vi "Initialise.vi"(8 "error in (no error)":errorcluster, 10 "Message in":refnum<class "InitialiseMessage.lvclass">, 11 "DAQMH121119OrcaFlash in":refnum<class "DAQOrcaFlash.lvclass">) -> (0 "error out":errorcluster, 3 "DAQMH121119OrcaFlash out":refnum<class "DAQOrcaFlash.lvclass">)   [LabVIEW 2012, in "DAQOrcaFlash.lvclass"]
doc: "This member function is called when the statemachine in the run.vi receives an 'initialise' message. It mainly initialises the RabbitMQ connectivity. \n\nOverride this member function in your derived class to initialise hardware or software resources (but don't forget to call the parent method). If your component owns subcomponents, they count as resources, so you have to initialise them by calling their own initialise functions."
uses:
  DAQOrcaFlash.lvclass
  <vilib>/Distrio/Murmex/InitialiseMessage/InitialiseMessage.lvclass
  <vilib>/Distrio/Murmex/Murmex/Murmex.lvclass
  <vilib>/Distrio/Murmex/TerminateMessage/TerminateMessage.lvclass
  <vilib>/Distrio/Murmex/UpdateMessage/UpdateMessage.lvclass
  imaging_mode.ctl
  DAQOrcaFlash.lvclass/DAQOrcaFlash.ctl
  <vilib>/Distrio/Murmex/GenericMessage/GenericMessage.lvclass
  <vilib>/Distrio/Murmex/Message/Add or replace parameter.vi
panel:
  # "This method is called when the INTIALISE\ntrigger is sent. \n\nOverride this method when your component needs to\nrespond to this trigger. \n\nCall parent for proper implementation"
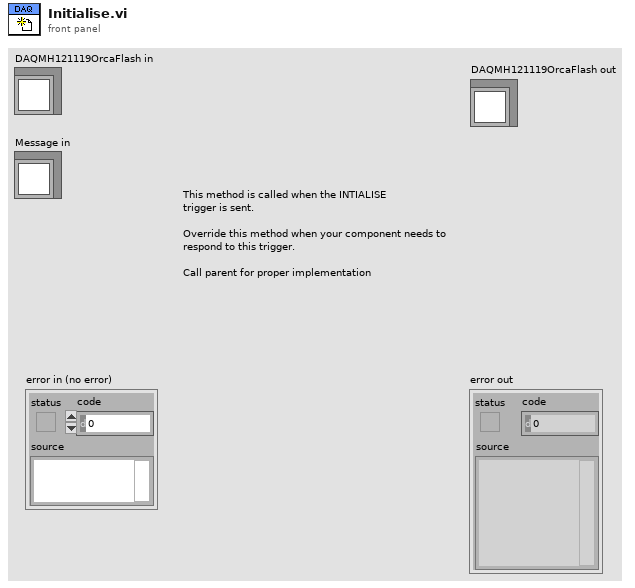
[diagram p1: front panel]
types:
  T1 = typedef "DAQOrcaFlash.lvclass/imaging_mode.ctl" = enum16{"focus mode", "single sweep"}
  T2 = cluster{"Mode":u32, "Polarity":u32, "Period":dbl, "Delay":dbl}
  T3 = typedef "Image Type" = u32
  T4 = typedef "IMAQ Image.ctl" = refnum<image>
  T5 = cluster{"height":u32, "width":u32, "datatype":u32}
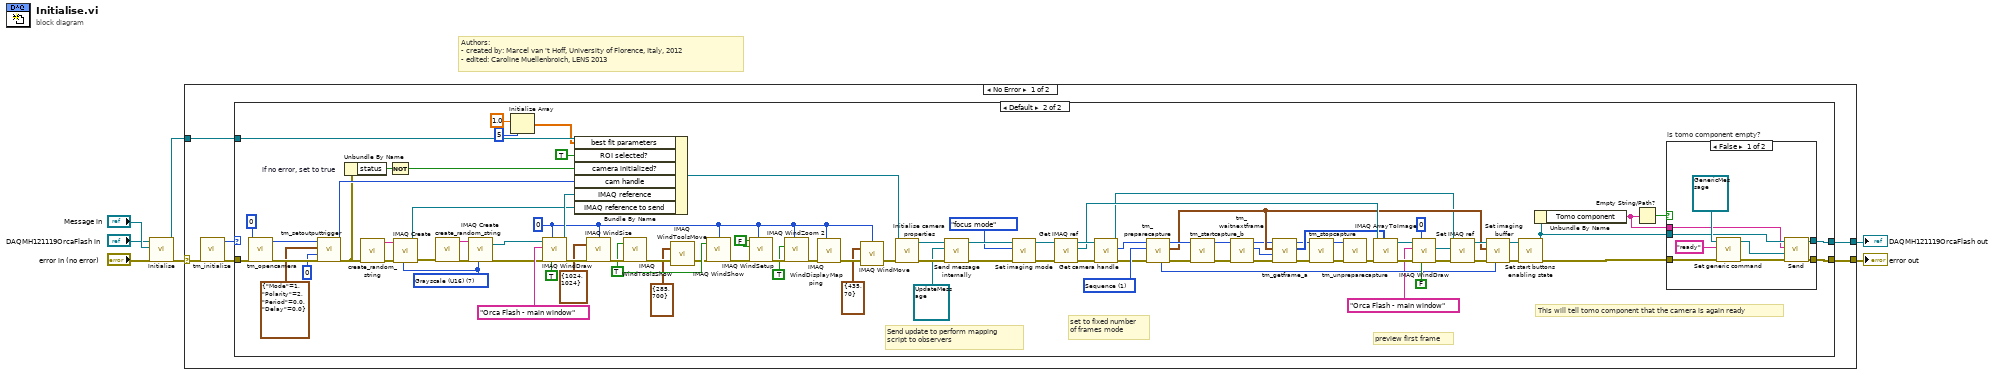
[diagram p0: block diagram]
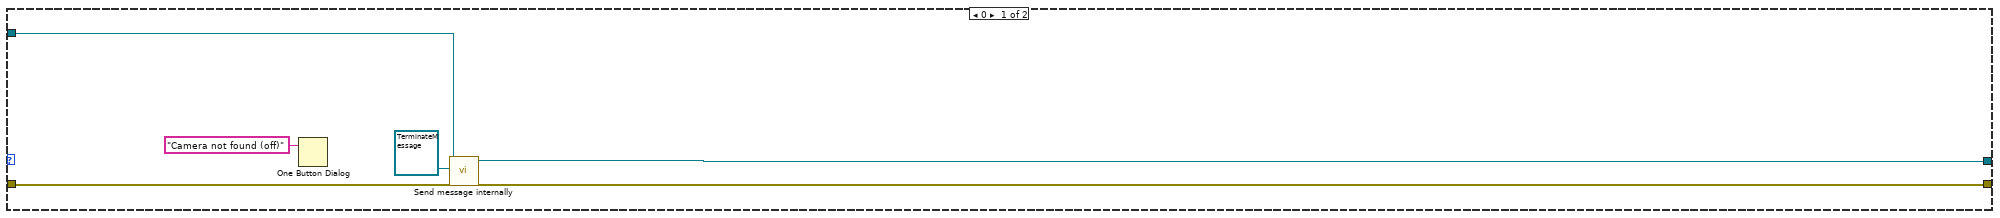
[diagram p2: hidden frame]
diagram:
  # "Authors: \n- created by: Marcel van 't Hoff, University of Florence, Italy, 2012\n- edited: Caroline Muellenbroich, LENS 2013"
  n1 = call-parent "Initialise.vi"("error in (no error)"="error in (no error)", "Message in"="Message in", "Murmex in"="DAQMH121119OrcaFlash in") -> ("error out"=w4:errorcluster, "Murmex out"=w3:refnum<class "DAQOrcaFlash.lvclass">)  [unwired: 7 in]
  n2 = case shown="No Error" w4 {
    selector: w4 -> [w12 w122]
    tunnel: w3 -> [w11 w123]
    tunnel: [w10 w123] -> w2
    tunnel: [w9 w122] -> w1
    frame No Error {
      n3 = call <userlib>:"tm_initialize.vi"("error in (no error)"=w12) -> ("error out"=w13:errorcluster, "Number Of Cameras"=w8:u32)  [unwired: 7 in, 2 out]
      n4 = case shown="Default" w8 {
        tunnel: w13 -> [w19 w110]
        tunnel: w11 -> [w17 w106]
        tunnel: [w16 w39] -> w10
        tunnel: [w18 w40] -> w9
        frame 0 {
          n5 = One Button Dialog(message="Camera not found (off)") -> ()  [unwired: 1 in, 1 out]
          n6 = call <vilib>:"Send message internally.vi"("error in (no error)"=w19, "Message"=refnum<class "TerminateMessage.lvclass"> refnum ("TerminateMessage"), "Murmex in"=w17) -> ("error out"=w18:errorcluster, "Murmex out"=w16:refnum<class "DAQOrcaFlash.lvclass">)  [unwired: 7 in]
        }
        frame Default {
          w68 = 1 items=["Snap", "Sequence"] ("Capture mode")
          w95 = FALSE ("Window can grow? (Yes)")
          w24 = 0 ("Window Number (0...15)")
          w97 = TRUE ("Hide/Show (Show)")
          w84 = T3 7 items=["Grayscale (U8)", "Grayscale (I16)", "Grayscale (SGL)", "Complex (CSG)", "RGB (U32)", "HSL (U32)", "RGB (U64)", "Grayscale (U16)"] ("Image Type")
          # "This will tell tomo component that the camera is again ready"
          # "preview first frame"
          # "set to fixed number\nof frames mode"
          # "Send update to perform mapping\nscript to observers"
          n7 = call <userlib>:"tm_opencamera.vi"("error in (no error)"=w110, "Camera Index"=u32 0) -> ("error out"=w91:errorcluster, "Handle out"=w92:u32)  [unwired: 7 in, 1 out]
          n8 = call <userlib>:"tm_setoutputtrigger.vi"("error in (no error)"=w91, "Index"=0, "Parameters"=T2 {"Mode"=1, "Polarity"=2, "Period"=0.0, "Delay"=0.0}, "Handle in"=w92) -> ("error out"=w78:errorcluster, "Handle out"=w88:u32)  [unwired: 6 in]
          n9 = Unbundle By Name "if no error, set to true"(w78) -> ("status"=w77:bool)
          n10 = call "create_random_string.vi"("error in (no error)"=w78) -> ("error out"=w85:errorcluster, "random string"=w83:string)  [unwired: 9 in]
          n11 = Not(x=w77) -> (.not. x?=w76:bool)
          n12 = call "IMAQ Create"("Image Name"=w83, "Image Type"=w84, "error in (no error)"=w85) -> ("New Image"=w82:T4, "error out"=w86:errorcluster)  [unwired: 2 in]
          n13 = call "create_random_string.vi"("error in (no error)"=w86) -> ("error out"=w108:errorcluster, "random string"=w107:string)  [unwired: 9 in]
          n14 = call "IMAQ Create"("Image Name"=w107, "Image Type"=w84, "error in (no error)"=w108) -> ("New Image"=w104:T4, "error out"=w101:errorcluster)  [unwired: 2 in]
          n15 = Initialize Array(1.0 ("element"), 5 ("dimension size")) -> (w33:dbl[])
          n16 = call "IMAQ WindDraw"("Resize to Image Size? (Y)"=TRUE, "Window Number (0...15)"=w24, "error in (no error)"=w101, "Title"="Orca Flash - main window", "Image"=w104) -> ("error out"=w100:errorcluster, "Image Out (duplicate)"=w105:T4)  [unwired: 5 in]
          n17 = Bundle By Name(cluster=w106, "best fit parameters"=w33, "ROI selected?"=TRUE ("Runtime cluster.ROI selected?"), "camera initialized?"=w76, "cam handle"=w88, "IMAQ reference"=w105, "IMAQ reference to send"=w82) -> (w87:refnum<class "DAQOrcaFlash.lvclass">)
          n18 = call "IMAQ WindSize"("error in (no error)"=w100, "Width & Height"=cluster{"Width":i32, "Height":i32} {"Width"=1024, "Height"=1024}, "Window Number"=w24) -> ("error out"=w99:errorcluster)  [unwired: 3 in, 2 out]
          n19 = call "IMAQ WindToolsShow"("Hide/Show (Show)"=w97, "error in (no error)"=w99) -> ("error out"=w22:errorcluster)  [unwired: 3 in, 1 out]
          n20 = call "IMAQ WindToolsMove"("Coordinates"=cluster{"X Position":i32, "Y Position":i32} {"X Position"=285, "Y Position"=700}, "error in (no error)"=w22) -> ("error out"=w21:errorcluster)  [unwired: 3 in, 1 out]
          n21 = call "IMAQ WindShow"("error in (no error)"=w21, "Hide/Show (Show)"=w97, "Window Number (0...15)"=w24) -> ("error out"=w96:errorcluster)  [unwired: 3 in, 2 out]
          n22 = call "IMAQ WindSetup"("Window Number (0...15)"=w24, "error in (no error)"=w96, "Window can close? (Yes)"=w95, "Window can grow? (Yes)"=w95) -> ("error out"=w94:errorcluster)  [unwired: 7 in]
          n23 = call "IMAQ WindZoom 2"("Window Number (0...15)"=w24, "error in (no error)"=w94, "Zoom to Fit? (False)"=TRUE) -> ("error out"=w75:errorcluster)  [unwired: 5 in, 3 out]
          n24 = call "IMAQ WindDisplayMapping"("Window Number (0...15)"=w24, "error in (no error)"=w75) -> ("error out"=w26:errorcluster)  [unwired: 8 in, 1 out]
          n25 = call "IMAQ WindMove"("Window Number (0...15)"=w24, "Coordinates (screen)"=cluster{"X Position":i32, "Y Position":i32} {"X Position"=435, "Y Position"=70}, "error in (no error)"=w26) -> ("error out"=w25:errorcluster)  [unwired: 2 in, 1 out]
          n26 = call-dynamic "Initialise camera properties.vi"("error in (no error)"=w25, "DAQOrcaFlash in"=w87) -> ("error out"=w81:errorcluster, "DAQOrcaFlash out"=w80:refnum<class "DAQOrcaFlash.lvclass">)  [unwired: 8 in]
          n27 = call <vilib>:"Send message internally.vi"("error in (no error)"=w81, "Message"=refnum<class "UpdateMessage.lvclass"> refnum ("Distrio Murmex 1.0:UpdateMessage"), "Murmex in"=w80) -> ("error out"=w44:errorcluster, "Murmex out"=w42:refnum<class "DAQOrcaFlash.lvclass">)  [unwired: 7 in]
          n28 = call "Set imaging mode.vi"("error in (no error)"=w44, "imaging mode"=imaging_mode."focus mode", "DAQMH121119OrcaFlash in"=w42) -> ("error out"=w45:errorcluster, "DAQMH121119OrcaFlash out"=w43:refnum<class "DAQOrcaFlash.lvclass">)  [unwired: 7 in]
          n29 = call "Get IMAQ ref.vi"("error in (no error)"=w45, "DAQMH121119OrcaFlash in"=w43) -> ("error out"=w73:errorcluster, "IMAQ reference"=w63:T4, "DAQMH121119OrcaFlash out"=w74:refnum<class "DAQOrcaFlash.lvclass">)  [unwired: 7 in]
          n30 = call "Get camera handle.vi"("error in (no error)"=w73, "DAQMH121119OrcaFlash in"=w74) -> ("error out"=w54:errorcluster, "cam handle"=w55:u32, "DAQMH121119OrcaFlash out"=w57:refnum<class "DAQOrcaFlash.lvclass">)  [unwired: 7 in]
          n31 = call <userlib>:"tm_preparecapture.vi"("error in (no error)"=w54, "Capture mode"=w68, "Handle in"=w55) -> ("error out"=w69:errorcluster, "Buffer Info"=w61:T5, "Handle out"=w67:u32, "Image type"=w60:u32)  [unwired: 5 in]
          n32 = call <userlib>:"tm_startcapture_b.vi"("error in (no error)"=w69, "Handle in"=w67) -> ("error out"=w66:errorcluster, "Handle out"=w46:u32)  [unwired: 8 in]
          n33 = call <userlib>:"tm_waitnextframe.vi"("error in (no error)"=w66, "Handle in"=w46) -> ("error out"=w53:errorcluster, "Frame Index"=w65:i32, "Handle out"=w52:u32)  [unwired: 6 in, 1 out]
          n34 = call <userlib>:"tm_getframe_a.vi"("error in (no error)"=w53, "Frame Index"=w65, "Buffer Info"=w61, "Handle in"=w52) -> ("error out"=w48:errorcluster, "Data 16"=w59:u16[][], "Handle out"=w51:u32)  [unwired: 3 in, 2 out]
          n35 = call <userlib>:"tm_stopcapture.vi"("error in (no error)"=w48, "Handle in"=w51) -> ("error out"=w49:errorcluster, "Handle out"=w50:u32)  [unwired: 8 in]
          n36 = call <userlib>:"tm_unpreparecapture.vi"("error in (no error)"=w49, "Handle in"=w50) -> ("error out"=w47:errorcluster)  [unwired: 8 in, 1 out]
          n37 = call "IMAQ ArrayToImage"("Image Pixels (U16)"=w59, "error in (no error)"=w47, "Image"=w63) -> ("error out"=w64:errorcluster, "Image Out"=w62:T4)  [unwired: 7 in]
          n38 = call "IMAQ WindDraw"("Resize to Image Size? (Y)"=FALSE, "Window Number (0...15)"=0, "error in (no error)"=w64, "Title"="Orca Flash - main window", "Image"=w62) -> ("error out"=w27:errorcluster, "Image Out (duplicate)"=w58:T4)  [unwired: 5 in]
          n39 = call "Set IMAQ ref.vi"("error in (no error)"=w27, "IMAQ reference"=w58, "DAQMH121119OrcaFlash in"=w57) -> ("error out"=w71:errorcluster, "DAQMH121119OrcaFlash out"=w72:refnum<class "DAQOrcaFlash.lvclass">)  [unwired: 7 in]
          n40 = call "Set imaging buffer.vi"("Image type"=w60, "error in (no error)"=w71, "Buffer"=w61, "DAQMH121119OrcaFlash in"=w72) -> ("error out"=w30:errorcluster, "DAQMH121119OrcaFlash out"=w32:refnum<class "DAQOrcaFlash.lvclass">)  [unwired: 6 in]
          n41 = call-dynamic "Set start buttons enabling state.vi"("error in (no error)"=w30, "DAQOrcaFlash in"=w32) -> ("error out"=w29:errorcluster, "DAQOrcaFlash out"=w31:refnum<class "DAQOrcaFlash.lvclass">)  [unwired: 8 in]
          n42 = Unbundle By Name(w31) -> ("Tomo component"=w37:string)
          n43 = Empty String/Path?(string/path=w37) -> (empty?=w38:bool)
          n44 = case "is tomo component empty?" shown="False" w38 {
            tunnel: w29 -> [w119 w120]
            tunnel: [w117 w120] -> w40
            tunnel: w31 -> [w113 w121]
            tunnel: [w112 w121] -> w39
            tunnel: w37 -> [w111 _]
            frame False {
              n45 = call <vilib>:"Set generic command.vi"("error in (no error)"=w119, "generic command"="ready", "GenericMessage in"=refnum<class "GenericMessage.lvclass"> refnum ("Distrio Murmex 1.5:GenericMessage")) -> ("error out"=w118:errorcluster, "GenericMessage out"=w114:refnum<class "GenericMessage.lvclass">)  [unwired: 7 in]
              n46 = call <vilib>:"Send.vi"("error in (no error)"=w118, "Message"=w114, "recipient"=w111, "Murmex in"=w113) -> ("error out"=w117:errorcluster, "Murmex out"=w112:refnum<class "DAQOrcaFlash.lvclass">)  [unwired: 6 in]
            }
            frame True {
            }
          }
        }
      }
    }
    frame Error {
    }
  }
  "error out" <- w1
  "DAQMH121119OrcaFlash out" <- w2
